vi "lab7-dac.vi"() -> ()   [LabVIEW 2018]
uses:
  <vilib>/DAQmx/write.llb/DAQmx Write (Analog 1D DBL 1Chan NSamp).vi
  <vilib>/DAQmx/create/channels.llb/DAQmx Create Channel (AO-Voltage-Basic).vi
  <vilib>/DAQmx/configure/timing.llb/DAQmx Timing (Sample Clock).vi
  <vilib>/DAQmx/miscellaneous.llb/DAQmx Fill In Error Info.vi
panel:
  in  "samples per channel":i32=1000
  in  "rate":dbl=1000.0 format="%0.2f"
  out "error out":errorcluster
  in  "error in":errorcluster
  in  "Amplitude":dbl
  in  "Number":i32
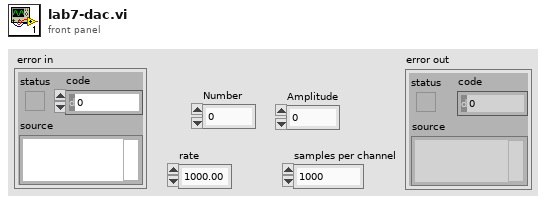
[diagram p1: front panel]
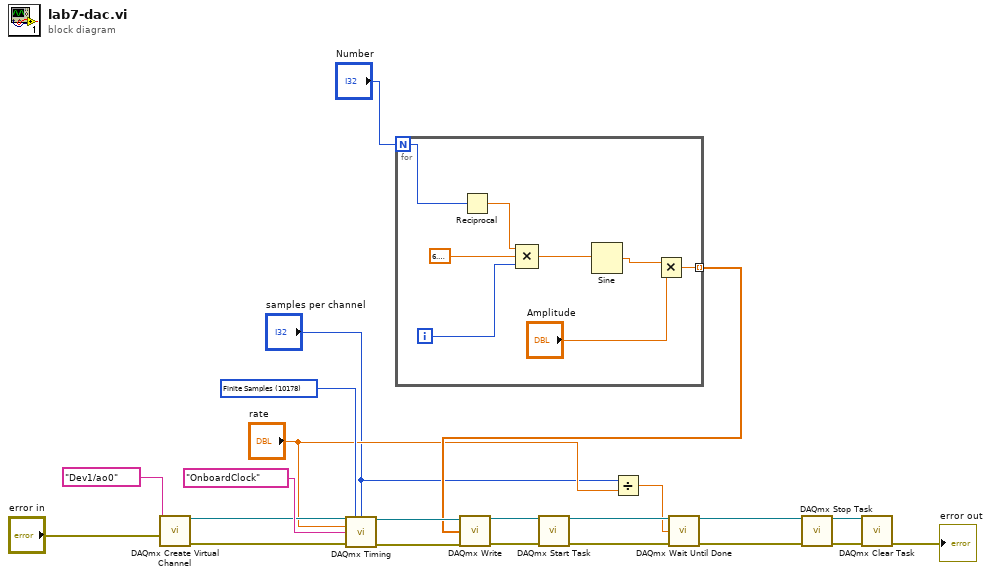
[diagram p0: block diagram]
diagram:
  w17 = 10178 items=["Finite Samples"=10178, "Continuous Samples"=10123, "Hardware Timed Single Point"=12522] ("sample mode")
  n1 = call-poly <vilib>:"DAQmx Create Virtual Channel.vi"("physical channels"=tag "Dev1/ao0", "error in"="error in") -> ("task out"=w16:refnum<k21>, "error out"=w15:errorcluster)  [unwired: 12 in]
  n2 = call-poly <vilib>:"DAQmx Timing.vi"("task/channels in"=w16, "sample mode"=w17, "samples per channel"="samples per channel", "rate"="rate", "source"=tag "OnboardClock", "error in"=w15) -> ("task out"=w14:refnum<k21>, "error out"=w13:errorcluster)  [unwired: 8 in]
  n3 = for {
    N: "Number" -> [w30]
    tunnel: [w23] -> w9 mode=indexing
    i -> [w27]
    n4 = Reciprocal(x=w30) -> (1/x=w29:dbl)
    n5 = Compound Arithmetic op=MULTIPLY(w29, 6.283185307179586, w27) -> (w26:dbl)
    n6 = Sine(x=w26) -> (sin(x)=w24:dbl)
    n7 = Multiply(x=w24, y="Amplitude") -> (x*y=w23:dbl)
  }
  n8 = call-poly <vilib>:"DAQmx Write.vi"("task/channels in"=w14, "data"=w9, "error in"=w13) -> ("task out"=w12:refnum<k21>, "error out"=w11:errorcluster)  [unwired: 10 in, 1 out]
  n9 = call <vilib>:"DAQmx Start Task.vi"("task/channels in"=w12, "error in"=w11) -> ("task out"=w8:refnum<k21>, "error out"=w6:errorcluster)  [unwired: 12 in]
  n10 = Divide(x="samples per channel", y="rate") -> (x/y=w3:dbl)
  n11 = call <vilib>:"DAQmx Wait Until Done.vi"("task/channels in"=w8, "timeout (sec)"=w3, "error in"=w6) -> ("task out"=w7:refnum<k21>, "error out"=w5:errorcluster)  [unwired: 11 in]
  n12 = call <vilib>:"DAQmx Stop Task.vi"("task/channels in"=w7, "error in"=w5) -> ("task out"=w21:refnum<k21>, "error out"=w20:errorcluster)  [unwired: 12 in]
  n13 = call <vilib>:"DAQmx Clear Task.vi"("task in"=w21, "error in"=w20) -> ("error out"=→"error out":errorcluster)  [unwired: 13 in]
